vi "PIO.vi"(3 "input":bool, 4 "channel":dbl=1.0 min=1.0 max=6.0, 5 "error in (no error)":errorcluster, 6 "VISA resource Input":refnum<visa-resource-name>) -> (0 "output":bool, 1 "error out":errorcluster, 2 "VISA resource Quit":refnum<visa-resource-name>)   [LabVIEW 2011]
panel:
  out "unsigned byte array":u8[](array[numeric])
  out "return count":u32
  out "Read Pio command":u8[](array[numeric])
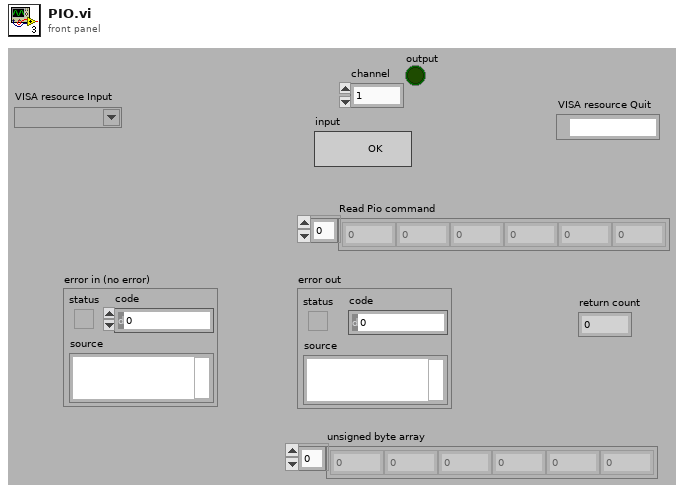
[diagram p1: front panel]
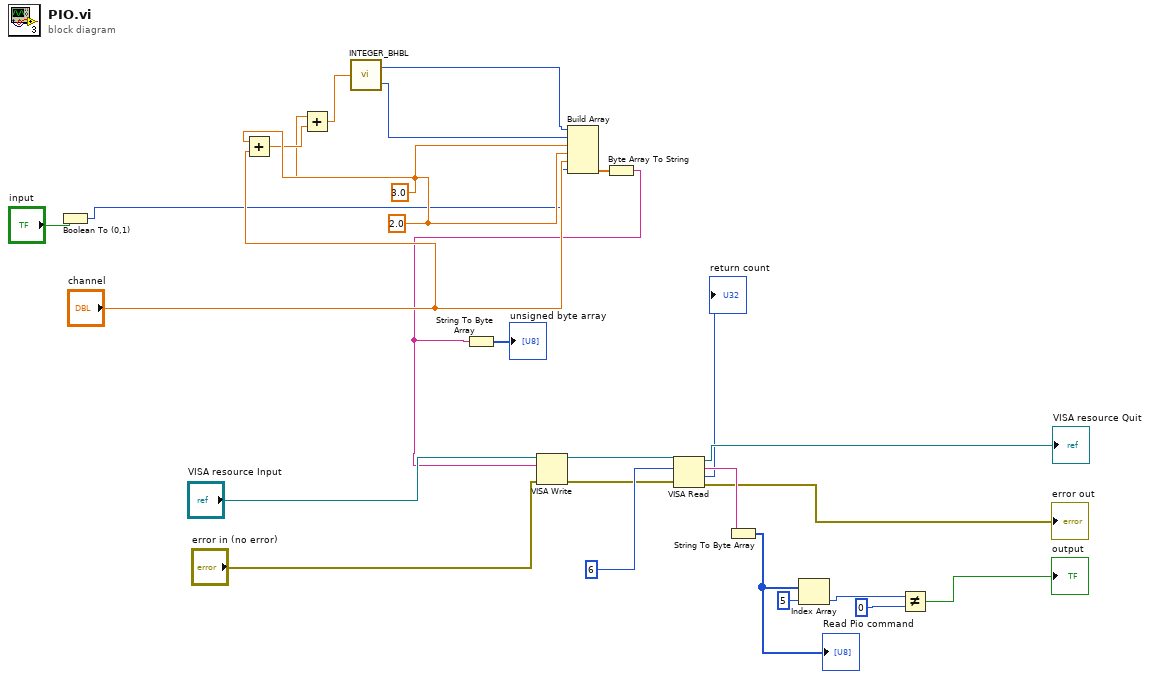
[diagram p0: block diagram]
diagram:
  w15 = 2.0 ("element")
  w13 = 3.0 ("element")
  n1 = Boolean To (0,1)(Boolean="input") -> (0, 1=w6:i16)
  n2 = Add(x=w15, y="channel") -> (x+y=w14:dbl)
  n3 = Add(x=w13, y=w14) -> (x+y=w12:dbl)
  n4 = call "INTEGER_BHBL.vi"("int16"=w12) -> ("Lvalue"=w10:u8, "HValue"=w11:u8)
  n5 = Build Array(w11, w10, w13, w15, "channel", w6) -> (w20:dbl[])
  n6 = Byte Array To String(unsigned byte array=w20) -> (string=w9:string)
  n7 = String To Byte Array(string=w9) -> (unsigned byte array=→"unsigned byte array":u8[])
  n8 = VISA Write(VISA resource name="VISA resource Input", write buffer=w9, error in (no error)="error in (no error)") -> (VISA resource name out=w21:refnum<visa-resource-name>, error out=w23:errorcluster)  [unwired: 1 out]
  n9 = VISA Read(VISA resource name=w21, byte count=u32 6, error in (no error)=w23) -> (VISA resource name out=→"VISA resource Quit":refnum<visa-resource-name>, read buffer=w25:string, return count=→"return count":u32, error out=→"error out":errorcluster)
  n10 = String To Byte Array(string=w25) -> (unsigned byte array=w5:u8[])
  "Read Pio command" <- w5
  n11 = Index Array(array=w5, index=5) -> (element=w3:u8)
  n12 = Not Equal?(x=w3, y=u8 0) -> (x != y?=→"output":bool)
